vi "emi_Get Debug Disp status.vi"(9 "error in (no error)":errorcluster) -> (8 "Debug Disp":bool, 10 "error out":errorcluster)   [LabVIEW 2011]
doc: "Checks wheter the application id closeing,"
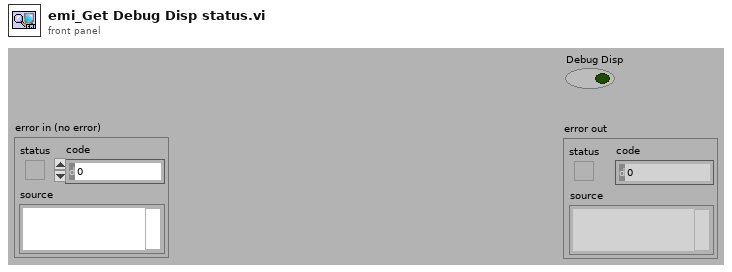
[diagram p1: front panel]
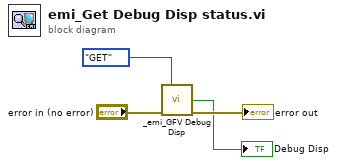
[diagram p0: block diagram]
diagram:
  n1 = call "_emi_GFV Debug Disp.vi"("Action(GET)"=enum16{"GET", "SET"}."GET", "error in (no error)"="error in (no error)") -> ("Debug Disp out"=→"Debug Disp":bool, "error out"=→"error out":errorcluster)  [unwired: 12 in]
